vi "Full Adder.vi"(9 "Input in":bool, 10 "Input 1":bool, 11 "Carry In":bool) -> (2 "Carry":bool, 3 "Sum":bool)   [LabVIEW 2018]
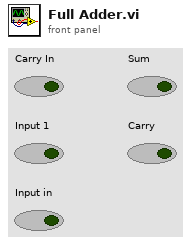
[diagram p1: front panel]
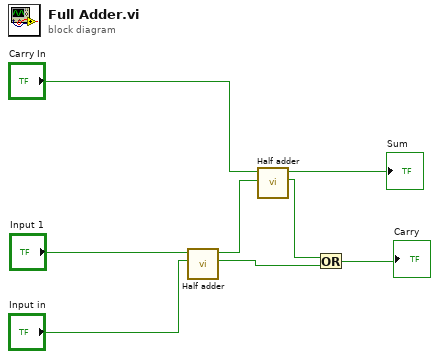
[diagram p0: block diagram]
diagram:
  n1 = call "Half adder.vi"("Input in"="Input in", "Input 1"="Input 1") -> ("Boolean"=w3:bool, "Boolean 2"=w6:bool)  [unwired: 8 in]
  n2 = call "Half adder.vi"("Input in"=w6, "Input 1"="Carry In") -> ("Boolean"=w4:bool, "Boolean 2"=→"Sum":bool)  [unwired: 8 in]
  n3 = Or(x=w4, y=w3) -> (x .or. y?=→"Carry":bool)
